vi "oauth2_authorize.vi"   [LabVIEW 2015, in "lv-dropbox.lvlib"]
uses:
  lv-dropbox.lvlib
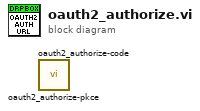
[diagram p0: block diagram]
diagram:
  n1 = call "oauth2_authorize-pkce.vi"() -> ()  [unwired: 10 in, 2 out]
  n2 = call "oauth2_authorize-code.vi"() -> ()  [unwired: 10 in, 2 out]
